vi "GVtdms.vi"() -> ()   [LabVIEW 2010]
panel:
  in  "TDMS-Datei":refnum<k34>
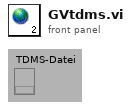
[diagram p1: front panel]
diagram:
